vi "white_ball_detect4_for_functionUse.vi"(1 "Circles":T1(array[cluster]), 2 "color_billard":T2) -> (0 "白球所在(已处理的)数组位置":i32)   [LabVIEW 2018]
uses:
  <vilib>/vision/Image Controls.llb/IMAQ Image.ctl
  <vilib>/vision/NI_Vision_Development_Module.lvlib
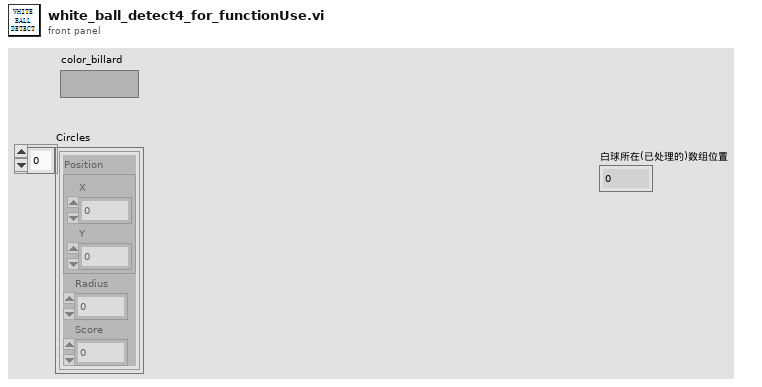
[diagram p1: front panel]
types:
  T1 = cluster{"Position":cluster{"X":sgl, "Y":sgl}, "Radius":dbl, "Score":dbl}[]
  T2 = typedef "IMAQ Image.ctl" = refnum<image>
  T3 = typedef "ROI Descriptor" = cluster{"Global Rectangle":i32[], "Contours":cluster{"ID":enum32{"External", "Internal"}, "Type":u32, "Coordinates":i32[]}[]}
  T4 = cluster{"Starting Value":sgl, "Incremental Value":sgl, "Histogram":u32[]}
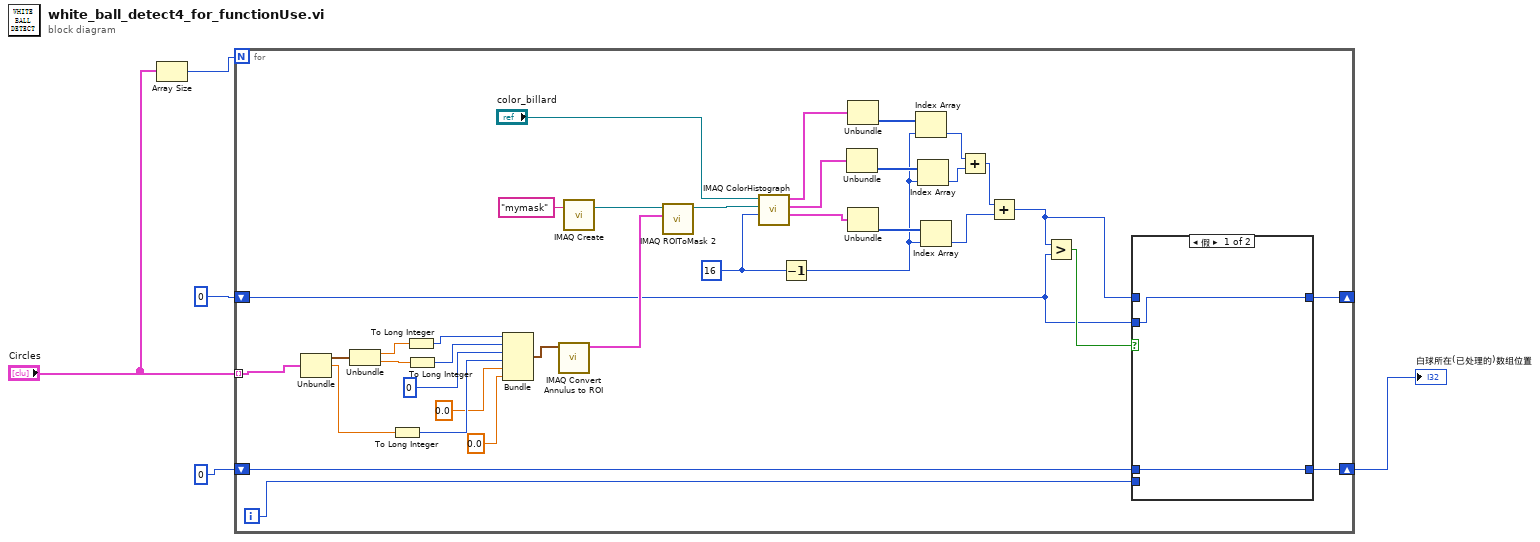
[diagram p0: block diagram]
diagram:
  n1 = Array Size(array="Circles") -> (size(s)=w5:i32)
  n2 = for {
    N: w5 -> [_]
    tunnel: "Circles" -> [w26] mode=indexing
    shift-right: [w11] -> _
    shift-left: 0 -> [w7]
    shift-right: [w8] -> w2
    shift-left: 0 -> [w10]
    i -> [w9]
    w19 = 16 ("Number of Classes")
    n3 = Unbundle(w26) -> ("Position"=w37:cluster{"X":sgl, "Y":sgl}, "Radius"=w34:dbl)  [unwired: 1 out]
    n4 = Unbundle(w37) -> ("X"=w36:sgl, "Y"=w35:sgl)
    n5 = To Long Integer(number=w34) -> (32bit integer=w30:i32)
    n6 = To Long Integer(number=w36) -> (32bit integer=w33:i32)
    n7 = To Long Integer(number=w35) -> (32bit integer=w32:i32)
    n8 = Bundle(w33, w32, 0, w30, 0.0, 0.0) -> (w27:cluster{i32, i32, i32, i32, dbl, dbl})  [unwired: 1 in]
    n9 = call "IMAQ Convert Annulus to ROI"("Annulus"=w27) -> ("ROI Descriptor"=w40:T3)  [unwired: 8 in, 1 out]
    n10 = call "IMAQ Create"("Image Name"="mymask") -> ("New Image"=w41:T2)  [unwired: 4 in, 1 out]
    n11 = call "IMAQ ROIToMask 2"("ROI Descriptor"=w40, "Image"=w41) -> ("Image Out"=w38:T2)  [unwired: 7 in, 2 out]
    n12 = call "IMAQ ColorHistograph"("Image Src"="color_billard", "Image Mask"=w38, "Number of Classes"=w19) -> ("Red or Hue Histogram Graph"=w25:T4, "Green or Sat Histogram Graph"=w24:T4, "Blue or Luma or Val or Inten Histogram Graph"=w23:T4)  [unwired: 3 in, 1 out]
    n13 = Decrement(x=w19) -> (x-1=w18:i32)
    n14 = Unbundle(w24) -> ("Histogram"=w21:u32[])  [unwired: 2 out]
    n15 = Unbundle(w25) -> ("Histogram"=w22:u32[])  [unwired: 2 out]
    n16 = Unbundle(w23) -> ("Histogram"=w20:u32[])  [unwired: 2 out]
    n17 = Index Array(array=w22, index=w18) -> (element=w17:u32)
    n18 = Index Array(array=w21, index=w18) -> (element=w16:u32)
    n19 = Index Array(array=w20, index=w18) -> (element=w15:u32)
    n20 = Add(x=w17, y=w16) -> (x+y=w14:u32)
    n21 = Add(x=w14, y=w15) -> (x+y=w12:u32)
    n22 = Greater?(x=w12, y=w7) -> (0:w13:bool)
    n23 = case shown="假" w13 {
      tunnel: w12 -> [_ w45]
      tunnel: [w43 w45] -> w11
      tunnel: w10 -> [w42 _]
      tunnel: w9 -> [_ w44]
      tunnel: [w42 w44] -> w8
      tunnel: w7 -> [w43 _]
      frame False {
      }
      frame True {
      }
    }
  }
  "白球所在(已处理的)数组位置" <- w2
